vi "User_Metadata.vi"() -> ()   [LabVIEW 2011]
uses:
  ADAM Controls/Channel_names.ctl
  ADAM Controls/Calib_type_ADAM.ctl
  Anemometry/Anemometry Sub Vis/Controls/Preference_Mode.ctl
  ADAM Controls/Channel_State.ctl
  ADAM Controls/Module_type_ADAM.ctl
  ADAM Controls/Update_scan_value.ctl
  Anemometry/Anemometry Sub Vis/Globals/Preference_global.vi
  Anemometry/Anemometry Sub Vis/Globals/Constants_global.vi
  Anemometry/Anemometry Sub Vis/Globals/Meas_global.vi
  Anemometry/Anemometry Sub Vis/Globals/Trav_pos_global.vi
panel:
  out "Channel Name 13":string
  out "Channel Name 12":string
  out "Channel Name 11":string
  in  "Value 13":string
  in  "Value 12":string
  in  "Value 11":string
  in  "Menu 13":u16(ring) items=["Edit Strings", "20mm Cubes"]
  in  "Menu 12":u16(ring) items=["Edit Strings", "20mm Cubes"]
  in  "Menu 11":u16(ring) items=["Edit Strings", "20mm Cubes"]
  in  "Edit Preference Panel":bool
  out "Rig Name":string="EnFlo Tunnel"
  in  "Edit Email Addresses":bool
  out "Email Addresses":string[](array[string])
  in  "Value 10":string
  in  "Value 9":string
  in  "Value 8":string
  in  "Value 7":string
  in  "Value 6":string
  in  "Menu 10":u16(ring) items=["Edit Strings", "20mm Cubes"]
  out "Channel Name 10":string
  in  "Menu 9":u16(ring) items=["Edit Strings", "None", "Ramp 29 x 390mm", "Ramp 9 x 175mm", "Rounded nose 18.2 x 55mm", "Rounded nose 9 x 150mm"]
  out "Channel Name 9":string
  in  "Menu 8":u16(ring) items=["Edit Strings", "20mm Cubes"]
  out "Channel Name 8":string
  in  "Menu 7":u16(ring) items=["Edit Strings", "0", "115", "65"]
  out "Channel Name 7":string
  in  "Menu 6":u16(ring) items=["Edit Strings", "0", "1", "16"]
  out "Channel Name 6":string
  out "Clear remaining channels":bool
  in  "Value 5":string
  in  "Menu 5":u16(ring) items=["Edit Strings", "0", "25", "6.25"]
  out "Channel Name 5":string
  in  "Value 4":string
  in  "Menu 4":u16(ring) items=["Edit Strings", "20 x 20mm", "40 x 40mm", "80 x 80mm", "None"]
  out "Channel Name 4":string
  in  "Value 3":string
  in  "Menu 3":u16(ring) items=["Edit Strings", "0", "10", "20", "Normal distribution with average = 10mm"]
  out "Channel Name 3":string
  in  "Value 2":string
  in  "Menu 2":u16(ring) items=["Edit Strings", "None", "Random blocks", "Uniform cube"]
  out "Channel Name 2":string
  in  "Modify User Channels":bool
  out "Channel No":i32
  out "First Loop":bool
  out "Index":i32
  in  "Value 1":string
  in  "Menu 1":u16(ring) items=["Edit Strings", "Aligned", "None", "Staggered"]
  out "Channel Name 1":string
  in  "stop":bool
  in  "OK":bool
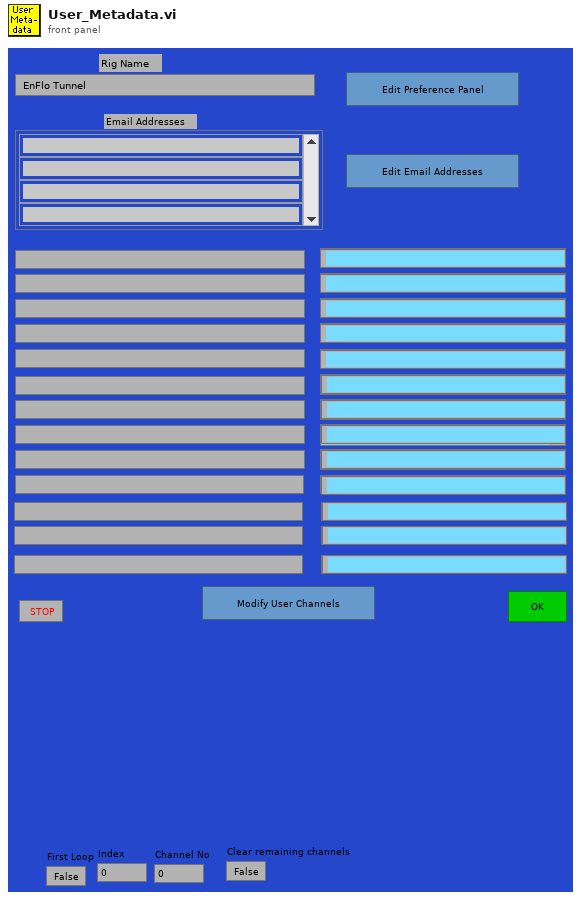
[diagram p1: front panel]
types:
  T1 = typedef "Channel_names.ctl" = enum16{"Active Only", "Active + Off", "All Channels"}
  T2 = typedef "Calib_type_ADAM.ctl" = enum16{"Raw", "Bx + A", "Cx^2 + Bx + A", "Dx^3 + Cx^2 + Bx + A", "In Band", "Hi-Tec Q", "Hi-Tec M_dot", "Text"}
  T3 = typedef "Preference_Mode.ctl" = enum16{"Load Preferences from file", "Save Preferences to file", "Load, Edit then Save"}
  T4 = typedef "Channel_State.ctl" = enum16{"On", "Off", "Always On", "Always Off"}
  T5 = typedef "Module_type_ADAM.ctl" = enum16{"4011", "4012", "4013", "4014", "4016", "4017", "4018", "4021", "4050", "4052", "4053", "4060", "4080", "5000", "5017", "5018", "5024", "5051", "5056", "5060", "6060", "Tracker", "WEST", "GILL", "JEM", "VICI", "Vaisala", "DRUCK", "Run VI Named:", "IR2100", "PPT", "Comparator", "VIRTUAL", "Hold Value", "Read A", "Read Ch", "Coded", "Client Info", "Web Client", "X10", "Test"}
  T6 = typedef "Ch_description_ADAM.ctl" = cluster{"Ch Name":string, "Type":T5, "Function":T7, "Ch State":T4, "Calibration type":T2, "A":dbl, "B":dbl, "C":dbl, "D":dbl, "Comments":string, "Address":T8, "String":string, "Duty":u16}
  T7 = typedef "Function_ADAM.ctl" = enum16{"Analogue Input", "Digital Input", "Event counter", "Event rate", "Analogue Output", "Digital Output", "Relay Output"}
  T8 = typedef "Address.ctl" = cluster{"Main":i32, "Ch.":i32, "Sub":i32, "Port Name":string}
  T9 = typedef "Update_scan_value.ctl" = cluster{"Channel Name":string, "New Value":dbl}
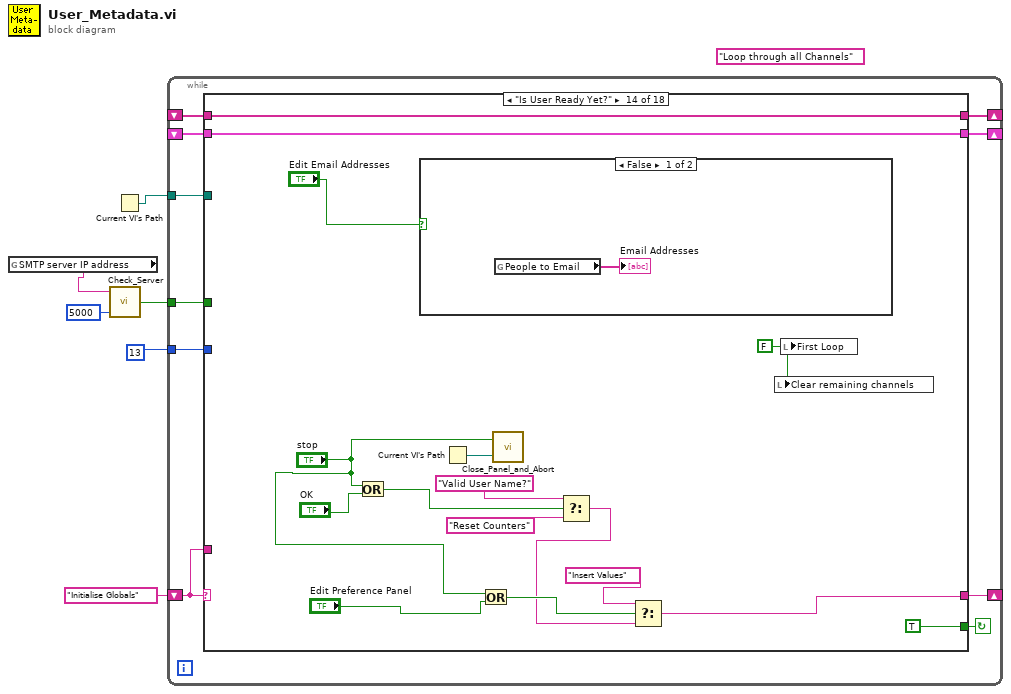
[diagram p0: block diagram]
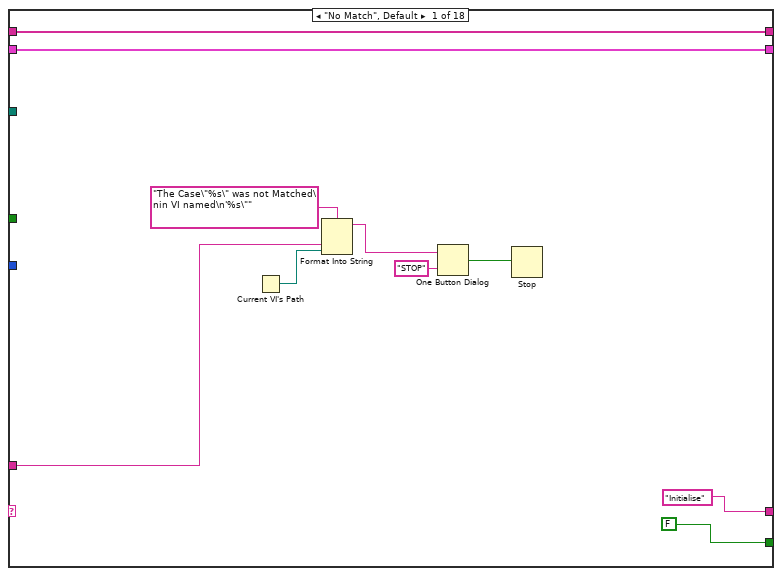
[diagram p2: hidden frame]
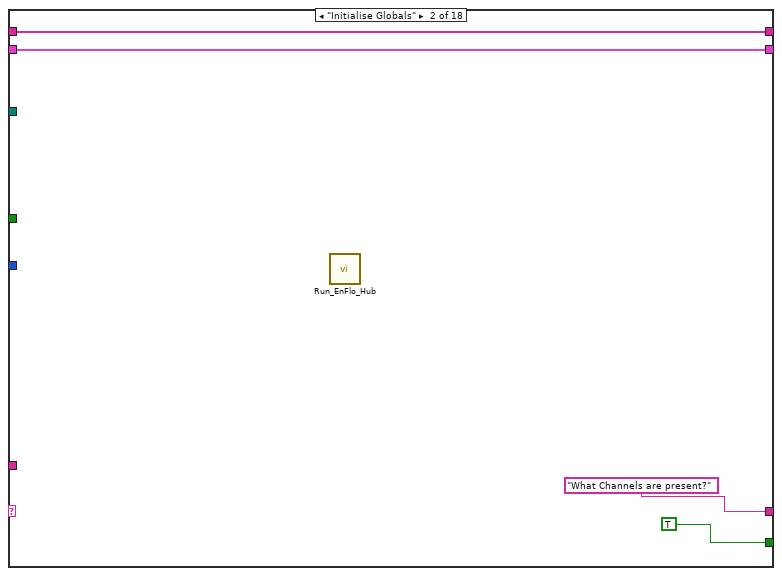
[diagram p3: hidden frame]
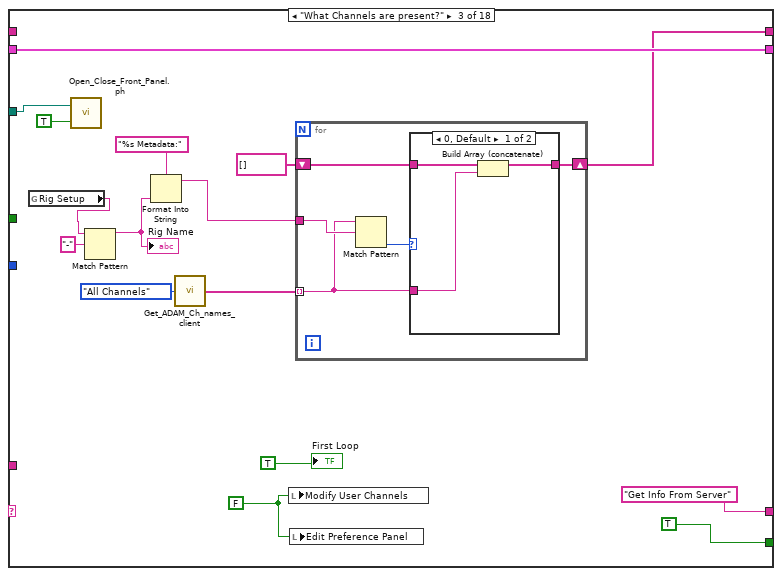
[diagram p4: hidden frame]
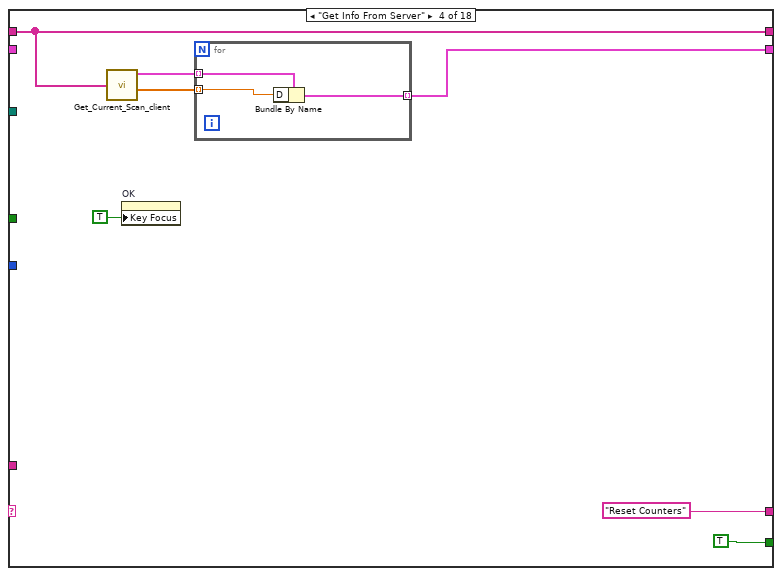
[diagram p6: hidden frame]
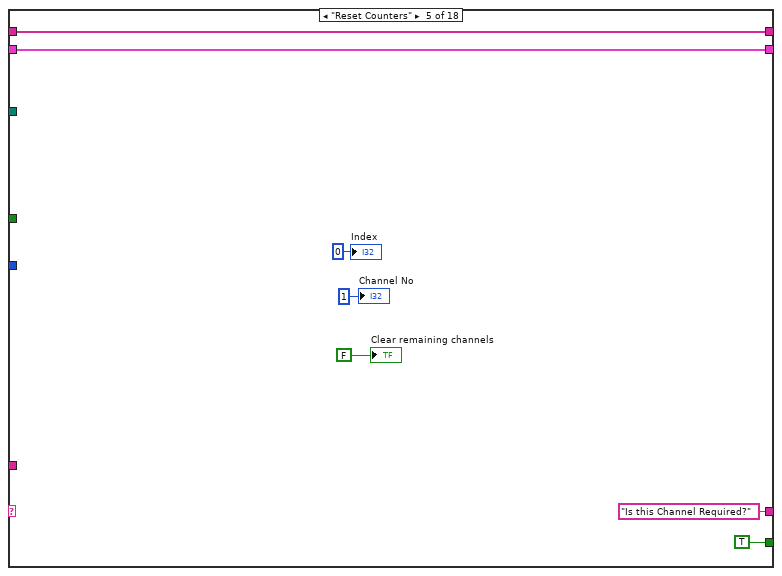
[diagram p7: hidden frame]
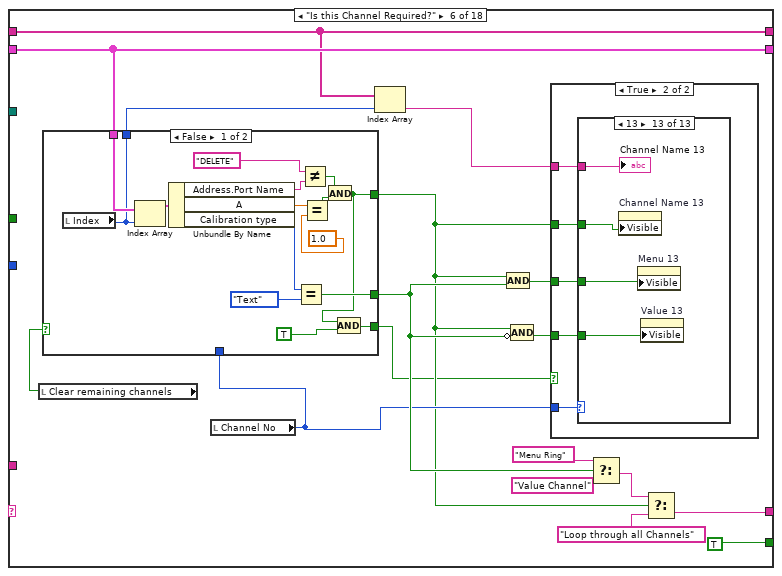
[diagram p8: hidden frame]
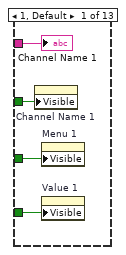
[diagram p10: hidden frame]
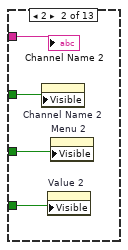
[diagram p11: hidden frame]
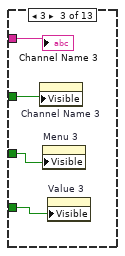
[diagram p12: hidden frame]
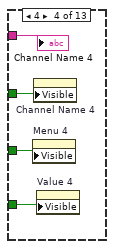
[diagram p13: hidden frame]
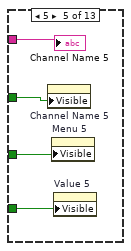
[diagram p14: hidden frame]
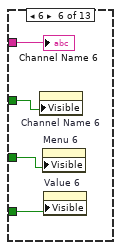
[diagram p15: hidden frame]
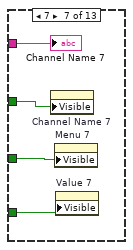
[diagram p16: hidden frame]
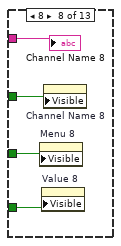
[diagram p17: hidden frame]
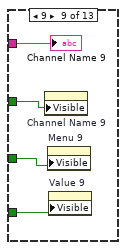
[diagram p18: hidden frame]
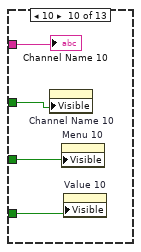
[diagram p19: hidden frame]
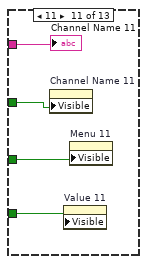
[diagram p20: hidden frame]
diagram:
  (unwired) "Loop through all Channels"
  n1 = global read "Preference_global.vi" "SMTP server IP address"() -> (w2:string)
  n2 = call "Check_Server.vi"("timeout ms (60000)"=5000, "address"=w2) -> ("OK"=w1:bool)  [unwired: 3 out]
  n3 = Current VI's Path() -> (path=w4:path)
  n4 = while {
    tunnel: 13 -> [w9]
    shift-left: _ -> [w12]
    shift-right: [w11] -> _
    shift-left: _ -> [w13]
    shift-right: [w14] -> _
    shift-left: "Initialise Globals" -> [w15]
    shift-right: [w10] -> _
    tunnel: w4 -> [w8]
    tunnel: w1 -> [w7]
    stop <- w16 continue-if-true
    n5 = case shown="\"Is User Ready Yet?\"" w15 {
      tunnel: [FALSE TRUE TRUE TRUE TRUE ("T button?") TRUE TRUE TRUE TRUE TRUE TRUE TRUE TRUE TRUE ("T button?") TRUE ("T button?") TRUE ("T button?") TRUE ("T button?") FALSE ("T button?")] -> w16
      tunnel: ["Initialise" "What Channels are present?" "Get Info From Server" "Reset Counters" "Is this Channel Required?" w84 w178 "Increment Channel No" "Increment Channel No" "Loop through all Channels" w398 "What Channels are present?" "Reset Counters" w447 "Insert Values" "Update Server" w489 "End"] -> w10
      tunnel: w15 -> [w21 _ _ _ _ _ _ _ _ _ _ _ _ _ _ _ _ _]
      tunnel: [w18 w28 w44 w57 w69 w88 w170 w305 w326 w396 w409 w430 w435 w457 w469 w477 w490 w537] -> w14
      tunnel: w13 -> [w18 w28 w44 _ w69 w88 w171 w304 w327 w396 w409 w430 w436 w457 w469 w475 w490 w537]
      tunnel: w12 -> [w17 w27 _ w60 w70 w78 w190 w309 w337 w395 w414 w431 _ w450 w467 w476 w491 w538]
      tunnel: [w17 w27 w40 w60 w70 w78 w190 w309 w337 w395 w414 w431 w434 w450 w467 w476 w491 w538] -> w11
      tunnel: w9 -> [_ _ _ _ _ _ _ _ _ _ w404 _ _ _ _ _ _ _]
      tunnel: w8 -> [_ _ w35 _ _ _ _ _ _ _ _ _ _ _ _ _ _ w535]
      tunnel: w7 -> [_ _ _ _ _ _ _ _ _ _ _ _ _ _ w462 _ _ _]
      frame "No Match", Default {
        n6 = Current VI's Path() -> (path=w20:path)
        n7 = Format Into String(format string="The Case\"%s\" was not Matched\nin VI named\n'%s\"" ("Format String"), w21, w20) -> (resulting string=w24:string)  [unwired: 2 in, 1 out]
        n8 = One Button Dialog(message=w24, button name ("OK")="STOP") -> (true=w22:bool)
        n9 = Stop(stop? (T)=w22) -> ()
      }
      frame "Initialise Globals" {
        n10 = call "Run_EnFlo_Hub.vi"() -> ()  [unwired: 8 out]
      }
      frame "What Channels are present?" {
        w34 = FALSE ("Add a New Channel")
        n11 = global read "Preference_global.vi" "Rig Setup"() -> (w32:string)
        n12 = call "Open_Close_Front_Panel.ph.vi"("Front Panel Window:Open"=TRUE, "VI path"=w35) -> ()  [unwired: 2 out]
        n13 = Match Pattern(string=w32, regular expression="-") -> (before substring=w31:string)  [unwired: 4 out]
        "Rig Name" <- w31
        n14 = Format Into String(format string="%s Metadata:" ("Format String"), w31) -> (resulting string=w37:string)  [unwired: 2 in, 1 out]
        n15 = call "Get_ADAM_Ch_names_client.vi"("Channel names set"=Channel_names."All Channels") -> ("Ch names"=w42:string[])
        n16 = local write "Modify User Channels"(w34) -> ()
        n17 = local write "Edit Preference Panel"(w34) -> ()
        n18 = for {
          tunnel: w37 -> [w51]
          tunnel: w42 -> [w49] mode=indexing
          shift-right: [w47] -> w40
          shift-left: string[] [] -> [w48]
          n19 = Match Pattern(string=w49, regular expression=w51) -> (offset past match=w50:i32)  [unwired: 4 out]
          n20 = case shown="0, Default" w50 {
            tunnel: w49 -> [w54 _]
            tunnel: w48 -> [w53 w55]
            tunnel: [w52 w55] -> w47
            frame 0, Default {
              n21 = Build Array (concatenate)(w53, w54) -> (w52:string[])
            }
            frame -1 {
            }
          }
        }
        "First Loop" <- TRUE ("First Loop")
      }
      frame "Get Info From Server" {
        n22 = call "Get_Current_Scan_client.vi"("ADAM Ch Names"=w60) -> ("Ch Description Array"=w59:T6[], "Numerical Values"=w58:dbl[])  [unwired: 2 out]
        n23 = property on="OK" class="Bool"("Key Focus"=TRUE) -> ()  [unwired: 2 in, 2 out]
        n24 = for {
          tunnel: w59 -> [w65] mode=indexing
          tunnel: w58 -> [w64] mode=indexing
          tunnel: [w63] -> w57 mode=indexing
          n25 = Bundle By Name(cluster=w65, "D"=w64) -> (w63:T6)
        }
      }
      frame "Reset Counters" {
        "Index" <- 0 ("Index")
        "Channel No" <- 1 ("Channel No")
        "Clear remaining channels" <- FALSE ("Clear remaining channels")
      }
      frame "Is this Channel Required?" {
        n26 = local read "Clear remaining channels"() -> (w76:bool)
        n27 = local read "Channel No"() -> (w75:i32)
        n28 = case shown="False" w76 {
          tunnel: w88 -> [w161 _]
          tunnel: [w147 w166] -> w74
          tunnel: [w157 w166] -> w83
          tunnel: [w156 0 ("Index")] -> w79
          tunnel: w75 -> [_ w163]
          tunnel: [w154 TRUE] -> w73
          frame False {
            n29 = local read "Index"() -> (w156:i32)
            n30 = Index Array(array=w161, index=w156) -> (element=w160:T6)
            n31 = Unbundle By Name(w160) -> ("Address.Port Name"=w151:string, "A"=w153:dbl, "Calibration type"=w158:T2)
            n32 = Equal?(x=w158, y=Calib_type_ADAM."Text" ("Calibration Type")) -> (x = y?=w157:bool)
            n33 = Not Equal?(x="DELETE", y=w151) -> (x != y?=w148:bool)
            n34 = Equal?(x=w153, y=1.0 ("x")) -> (x = y?=w149:bool)
            n35 = And(x=w148, y=w149) -> (x .and. y?=w147:bool)
            n36 = Compound Arithmetic op=AND(w147, TRUE ("Input")) -> (w154:bool)
          }
          frame True {
            w166 = FALSE
            n37 = Increment(x=w163) -> (x+1=w164:i32)
            n38 = local write "Channel No"(w164) -> ()
          }
        }
        n39 = Index Array(array=w78, index=w79) -> (element=w77:string)
        n40 = Compound Arithmetic op=AND(w74, w83) -> (w86:bool)
        n41 = Compound Arithmetic op=AND(w74, invert w83) -> (w87:bool)
        n42 = case shown="True" w73 {
          tunnel: w87 -> [_ w94]
          tunnel: w86 -> [_ w93]
          tunnel: w74 -> [_ w92]
          tunnel: w77 -> [_ w91]
          tunnel: w75 -> [_ w90]
          frame False {
          }
          frame True {
            n43 = case shown="13" w90 {
              tunnel: w92 -> [w96 w100 w104 w108 w112 w117 w121 w125 w129 w133 w138 w142 w146]
              tunnel: w94 -> [w98 w102 w106 w110 w114 w115 w119 w123 w127 w131 w135 w139 w143]
              tunnel: w93 -> [w97 w101 w105 w109 w113 w116 w120 w124 w128 w134 w136 w140 w144]
              tunnel: w91 -> [w95 w99 w103 w107 w111 w118 w122 w126 w130 w132 w137 w141 w145]
              frame 1, Default {
                n44 = property on="Channel Name 1" class="Str"("Visible"=w96) -> ()  [unwired: 2 in, 2 out]
                n45 = property on="Menu 1" class="Ring (strict)"("Visible"=w97) -> ()  [unwired: 2 in, 2 out]
                n46 = property on="Value 1" class="Str"("Visible"=w98) -> ()  [unwired: 2 in, 2 out]
                "Channel Name 1" <- w95
              }
              frame 2 {
                n47 = property on="Channel Name 2" class="Str"("Visible"=w100) -> ()  [unwired: 2 in, 2 out]
                n48 = property on="Value 2" class="Str"("Visible"=w102) -> ()  [unwired: 2 in, 2 out]
                n49 = property on="Menu 2" class="Ring (strict)"("Visible"=w101) -> ()  [unwired: 2 in, 2 out]
                "Channel Name 2" <- w99
              }
              frame 3 {
                n50 = property on="Channel Name 3" class="Str"("Visible"=w104) -> ()  [unwired: 2 in, 2 out]
                n51 = property on="Menu 3" class="Ring (strict)"("Visible"=w105) -> ()  [unwired: 2 in, 2 out]
                n52 = property on="Value 3" class="Str"("Visible"=w106) -> ()  [unwired: 2 in, 2 out]
                "Channel Name 3" <- w103
              }
              frame 4 {
                n53 = property on="Menu 4" class="Ring (strict)"("Visible"=w109) -> ()  [unwired: 2 in, 2 out]
                n54 = property on="Channel Name 4" class="Str"("Visible"=w108) -> ()  [unwired: 2 in, 2 out]
                n55 = property on="Value 4" class="Str"("Visible"=w110) -> ()  [unwired: 2 in, 2 out]
                "Channel Name 4" <- w107
              }
              frame 5 {
                n56 = property on="Channel Name 5" class="Str"("Visible"=w112) -> ()  [unwired: 2 in, 2 out]
                n57 = property on="Menu 5" class="Ring (strict)"("Visible"=w113) -> ()  [unwired: 2 in, 2 out]
                n58 = property on="Value 5" class="Str"("Visible"=w114) -> ()  [unwired: 2 in, 2 out]
                "Channel Name 5" <- w111
              }
              frame 6 {
                n59 = property on="Channel Name 6" class="Str"("Visible"=w117) -> ()  [unwired: 2 in, 2 out]
                n60 = property on="Menu 6" class="Ring (strict)"("Visible"=w116) -> ()  [unwired: 2 in, 2 out]
                n61 = property on="Value 6" class="Str"("Visible"=w115) -> ()  [unwired: 2 in, 2 out]
                "Channel Name 6" <- w118
              }
              frame 7 {
                n62 = property on="Channel Name 7" class="Str"("Visible"=w121) -> ()  [unwired: 2 in, 2 out]
                n63 = property on="Menu 7" class="Ring (strict)"("Visible"=w120) -> ()  [unwired: 2 in, 2 out]
                n64 = property on="Value 7" class="Str"("Visible"=w119) -> ()  [unwired: 2 in, 2 out]
                "Channel Name 7" <- w122
              }
              frame 8 {
                n65 = property on="Menu 8" class="Ring (strict)"("Visible"=w124) -> ()  [unwired: 2 in, 2 out]
                n66 = property on="Value 8" class="Str"("Visible"=w123) -> ()  [unwired: 2 in, 2 out]
                n67 = property on="Channel Name 8" class="Str"("Visible"=w125) -> ()  [unwired: 2 in, 2 out]
                "Channel Name 8" <- w126
              }
              frame 9 {
                n68 = property on="Channel Name 9" class="Str"("Visible"=w129) -> ()  [unwired: 2 in, 2 out]
                n69 = property on="Menu 9" class="Ring (strict)"("Visible"=w128) -> ()  [unwired: 2 in, 2 out]
                n70 = property on="Value 9" class="Str"("Visible"=w127) -> ()  [unwired: 2 in, 2 out]
                "Channel Name 9" <- w130
              }
              frame 10 {
                n71 = property on="Channel Name 10" class="Str"("Visible"=w133) -> ()  [unwired: 2 in, 2 out]
                n72 = property on="Menu 10" class="Ring (strict)"("Visible"=w134) -> ()  [unwired: 2 in, 2 out]
                n73 = property on="Value 10" class="Str"("Visible"=w131) -> ()  [unwired: 2 in, 2 out]
                "Channel Name 10" <- w132
              }
              frame 11 {
                n74 = property on="Channel Name 11" class="Str"("Visible"=w138) -> ()  [unwired: 2 in, 2 out]
                n75 = property on="Value 11" class="Str"("Visible"=w135) -> ()  [unwired: 2 in, 2 out]
                n76 = property on="Menu 11" class="Ring (strict)"("Visible"=w136) -> ()  [unwired: 2 in, 2 out]
                "Channel Name 11" <- w137
              }
              frame 12 {
                n77 = property on="Channel Name 12" class="Str"("Visible"=w142) -> ()  [unwired: 2 in, 2 out]
                n78 = property on="Menu 12" class="Ring (strict)"("Visible"=w140) -> ()  [unwired: 2 in, 2 out]
                n79 = property on="Value 12" class="Str"("Visible"=w139) -> ()  [unwired: 2 in, 2 out]
                "Channel Name 12" <- w141
              }
              frame 13 {
                n80 = property on="Channel Name 13" class="Str"("Visible"=w146) -> ()  [unwired: 2 in, 2 out]
                n81 = property on="Menu 13" class="Ring (strict)"("Visible"=w144) -> ()  [unwired: 2 in, 2 out]
                n82 = property on="Value 13" class="Str"("Visible"=w143) -> ()  [unwired: 2 in, 2 out]
                "Channel Name 13" <- w145
              }
            }
          }
        }
        n83 = Select(t="Menu Ring", s=w83, f="Value Channel") -> (s? t:f=w81:string)
        n84 = Select(t=w81, s=w74, f="Loop through all Channels") -> (s? t:f=w84:string)
      }
      frame "Menu Ring" {
        n85 = local read "First Loop"() -> (w188:bool)
        n86 = local read "Index"() -> (w183:i32)
        n87 = Index Array(array=w171, index=w183) -> (element=w168:T6)
        n88 = Unbundle By Name(w168) -> ("String"=w189:string, "D"=w172:dbl)
        n89 = call "Get_array_values_fr_String.vi"("String Value"=w189) -> ("String array"=w176:string[])  [unwired: 1 out]
        n90 = To Unsigned Word Integer(number=w172) -> (unsigned 16bit integer=w187:u16)
        n91 = local read "Channel No"() -> (w182:i32)
        n92 = Build Array (concatenate)("Edit Strings", w176) -> (w177:string[])
        n93 = Increment(x=w187) -> (x+1=w185:u16)
        n94 = Array Size(array=w176) -> (size(s)=w175:i32)
        n95 = To Unsigned Word Integer(number=w175) -> (unsigned 16bit integer=w174:u16)
        n96 = case shown="13" w182 {
          tunnel: w188 -> [w198 w207 w215 w223 w231 w239 w247 w255 w263 w271 w279 w287 w295]
          tunnel: w185 -> [w197 w206 w214 w222 w230 w238 w246 w254 w262 w270 w278 w286 w294]
          tunnel: [w192 w202 w210 w218 w226 w234 w242 w250 w258 w266 w274 w282 w290] -> w184
          tunnel: w177 -> [w196 w200 w209 w217 w225 w232 w241 w249 w257 w265 w273 w281 w289]
          tunnel: w174 -> [w193 w203 w211 w219 w227 w235 w243 w251 w259 w267 w275 w283 w291]
          frame 1, Default {
            n97 = property on="Menu 1" class="Ring (strict)"("Strings []"=w196) -> ()  [unwired: 2 in, 2 out]
            n98 = Select(t=w197, s=w198, f="Menu 1") -> (s? t:f=w194:u16)
            n99 = Less?(x=w194, y=w193) -> (x < y?=w195:bool)
            n100 = Select(t=w194, s=w195, f=w193) -> (s? t:f=w192:u16)
            n101 = local write "Menu 1"(w192) -> ()
          }
          frame 2 {
            n102 = property on="Menu 2" class="Ring (strict)"("Strings []"=w200) -> ()  [unwired: 2 in, 2 out]
            n103 = Select(t=w206, s=w207, f="Menu 2") -> (s? t:f=w204:u16)
            n104 = Less?(x=w204, y=w203) -> (x < y?=w205:bool)
            n105 = Select(t=w204, s=w205, f=w203) -> (s? t:f=w202:u16)
            n106 = local write "Menu 2"(w202) -> ()
          }
          frame 3 {
            n107 = property on="Menu 3" class="Ring (strict)"("Strings []"=w209) -> ()  [unwired: 2 in, 2 out]
            n108 = Select(t=w214, s=w215, f="Menu 3") -> (s? t:f=w212:u16)
            n109 = Less?(x=w212, y=w211) -> (x < y?=w213:bool)
            n110 = Select(t=w212, s=w213, f=w211) -> (s? t:f=w210:u16)
            n111 = local write "Menu 3"(w210) -> ()
          }
          frame 4 {
            n112 = property on="Menu 4" class="Ring (strict)"("Strings []"=w217) -> ()  [unwired: 2 in, 2 out]
            n113 = Select(t=w222, s=w223, f="Menu 4") -> (s? t:f=w220:u16)
            n114 = Less?(x=w220, y=w219) -> (x < y?=w221:bool)
            n115 = Select(t=w220, s=w221, f=w219) -> (s? t:f=w218:u16)
            n116 = local write "Menu 4"(w218) -> ()
          }
          frame 5 {
            n117 = property on="Menu 5" class="Ring (strict)"("Strings []"=w225) -> ()  [unwired: 2 in, 2 out]
            n118 = Select(t=w230, s=w231, f="Menu 5") -> (s? t:f=w228:u16)
            n119 = Less?(x=w228, y=w227) -> (x < y?=w229:bool)
            n120 = Select(t=w228, s=w229, f=w227) -> (s? t:f=w226:u16)
            n121 = local write "Menu 5"(w226) -> ()
          }
          frame 6 {
            n122 = property on="Menu 6" class="Ring (strict)"("Strings []"=w232) -> ()  [unwired: 2 in, 2 out]
            n123 = Select(t=w238, s=w239, f="Menu 6") -> (s? t:f=w236:u16)
            n124 = Less?(x=w236, y=w235) -> (x < y?=w237:bool)
            n125 = Select(t=w236, s=w237, f=w235) -> (s? t:f=w234:u16)
            n126 = local write "Menu 6"(w234) -> ()
          }
          frame 7 {
            n127 = property on="Menu 7" class="Ring (strict)"("Strings []"=w241) -> ()  [unwired: 2 in, 2 out]
            n128 = Select(t=w246, s=w247, f="Menu 7") -> (s? t:f=w244:u16)
            n129 = Less?(x=w244, y=w243) -> (x < y?=w245:bool)
            n130 = Select(t=w244, s=w245, f=w243) -> (s? t:f=w242:u16)
            n131 = local write "Menu 7"(w242) -> ()
          }
          frame 8 {
            n132 = property on="Menu 8" class="Ring (strict)"("Strings []"=w249) -> ()  [unwired: 2 in, 2 out]
            n133 = Select(t=w254, s=w255, f="Menu 8") -> (s? t:f=w252:u16)
            n134 = Less?(x=w252, y=w251) -> (x < y?=w253:bool)
            n135 = Select(t=w252, s=w253, f=w251) -> (s? t:f=w250:u16)
            n136 = local write "Menu 8"(w250) -> ()
          }
          frame 9 {
            n137 = property on="Menu 9" class="Ring (strict)"("Strings []"=w257) -> ()  [unwired: 2 in, 2 out]
            n138 = Select(t=w262, s=w263, f="Menu 9") -> (s? t:f=w260:u16)
            n139 = Less?(x=w260, y=w259) -> (x < y?=w261:bool)
            n140 = Select(t=w260, s=w261, f=w259) -> (s? t:f=w258:u16)
            n141 = local write "Menu 9"(w258) -> ()
          }
          frame 10 {
            n142 = property on="Menu 10" class="Ring (strict)"("Strings []"=w265) -> ()  [unwired: 2 in, 2 out]
            n143 = Select(t=w270, s=w271, f="Menu 10") -> (s? t:f=w268:u16)
            n144 = Less?(x=w268, y=w267) -> (x < y?=w269:bool)
            n145 = Select(t=w268, s=w269, f=w267) -> (s? t:f=w266:u16)
            n146 = local write "Menu 10"(w266) -> ()
          }
          frame 11 {
            n147 = property on="Menu 11" class="Ring (strict)"("Strings []"=w273) -> ()  [unwired: 2 in, 2 out]
            n148 = Select(t=w278, s=w279, f="Menu 11") -> (s? t:f=w276:u16)
            n149 = Less?(x=w276, y=w275) -> (x < y?=w277:bool)
            n150 = Select(t=w276, s=w277, f=w275) -> (s? t:f=w274:u16)
            n151 = local write "Menu 11"(w274) -> ()
          }
          frame 12 {
            n152 = property on="Menu 12" class="Ring (strict)"("Strings []"=w281) -> ()  [unwired: 2 in, 2 out]
            n153 = Select(t=w286, s=w287, f="Menu 12") -> (s? t:f=w284:u16)
            n154 = Less?(x=w284, y=w283) -> (x < y?=w285:bool)
            n155 = Select(t=w284, s=w285, f=w283) -> (s? t:f=w282:u16)
            n156 = local write "Menu 12"(w282) -> ()
          }
          frame 13 {
            n157 = property on="Menu 13" class="Ring (strict)"("Strings []"=w289) -> ()  [unwired: 2 in, 2 out]
            n158 = Select(t=w294, s=w295, f="Menu 13") -> (s? t:f=w292:u16)
            n159 = Less?(x=w292, y=w291) -> (x < y?=w293:bool)
            n160 = Select(t=w292, s=w293, f=w291) -> (s? t:f=w290:u16)
            n161 = local write "Menu 13"(w290) -> ()
          }
        }
        n162 = Equal To 0?(x=w184) -> (x = 0?=w181:bool)
        n163 = Select(t="Edit Menu Strings", s=w181, f="Increment Channel No") -> (s? t:f=w178:string)
        n164 = Decrement(x=w184) -> (x-1=w173:u16)
        n165 = To Double Precision Float(number=w173) -> (double precision float=w169:dbl)
        n166 = Bundle By Name(cluster=w168, "D"=w169) -> (w167:T6)
        n167 = Replace Array Subset(array=w171, new element=w167, index=w183) -> (w170:T6[])
      }
      frame "Edit Menu Strings" {
        n168 = local read "Index"() -> (w299:i32)
        n169 = Index Array(array=w304, index=w299) -> (element=w308:T6)
        n170 = Unbundle By Name(w308) -> ("String"=w310:string, "Ch Name"=w298:string)
        n171 = call "Get_array_values_fr_String.vi"("String Value"=w310) -> ("String array"=w303:string[])  [unwired: 1 out]
        n172 = call "Edit_String_Options_list.vi"("Channel Name"=w298, "String array"=w303) -> ("New Selection Index"=w296:i32, "String array Out"=w302:string[])
        n173 = call "Put_Array_into_String.vi"("String array"=w302) -> ("String Value"=w307:string)
        n174 = local read "Channel No"() -> (w301:i32)
        n175 = Increment(x=w296) -> (x+1=w300:i32)
        n176 = Bundle By Name(cluster=w308, "String"=w307, "D"=w296) -> (w306:T6)
        n177 = To Unsigned Word Integer(number=w300) -> (unsigned 16bit integer=w297:u16)
        n178 = case shown="1, Default" w301 {
          tunnel: w297 -> [w313 w314 w315 w316 w317 w318 w319 w320 w321 w322 w323 w324 w325]
          frame 1, Default {
            n179 = local write "Menu 1"(w313) -> ()
          }
          frame 2 {
            n180 = local write "Menu 2"(w314) -> ()
          }
          frame 3 {
            n181 = local write "Menu 3"(w315) -> ()
          }
          frame 4 {
            n182 = local write "Menu 4"(w316) -> ()
          }
          frame 5 {
            n183 = local write "Menu 5"(w317) -> ()
          }
          frame 6 {
            n184 = local write "Menu 6"(w318) -> ()
          }
          frame 7 {
            n185 = local write "Menu 7"(w319) -> ()
          }
          frame 8 {
            n186 = local write "Menu 8"(w320) -> ()
          }
          frame 9 {
            n187 = local write "Menu 9"(w321) -> ()
          }
          frame 10 {
            n188 = local write "Menu 10"(w322) -> ()
          }
          frame 11 {
            n189 = local write "Menu 11"(w323) -> ()
          }
          frame 12 {
            n190 = local write "Menu 12"(w324) -> ()
          }
          frame 13 {
            n191 = local write "Menu 13"(w325) -> ()
          }
        }
        n192 = Replace Array Subset(array=w304, new element=w306, index=w299) -> (w305:T6[])
      }
      frame "Value Channel" {
        n193 = local read "Index"() -> (w336:i32)
        n194 = local read "First Loop"() -> (w334:bool)
        n195 = Index Array(array=w327, index=w336) -> (element=w328:T6)
        n196 = local read "Channel No"() -> (w335:i32)
        n197 = Unbundle By Name(w328) -> ("D"=w330:dbl)
        n198 = call "Number_2_string.vi"("number"=w330) -> ("String"=w333:string)  [unwired: 1 in]
        n199 = case shown="1, Default" w335 {
          tunnel: w334 -> [w343 w347 w351 w355 w359 w363 w367 w371 w375 w379 w383 w387 w391]
          tunnel: w333 -> [w342 w346 w350 w354 w358 w362 w366 w370 w374 w378 w382 w386 w390]
          tunnel: [w340 w345 w349 w353 w357 w361 w365 w369 w373 w377 w381 w385 w389] -> w332
          frame 1, Default {
            n200 = Select(t=w342, s=w343, f="Value 1") -> (s? t:f=w340:string)
            n201 = local write "Value 1"(w340) -> ()
          }
          frame 2 {
            n202 = Select(t=w346, s=w347, f="Value 2") -> (s? t:f=w345:string)
            n203 = local write "Value 2"(w345) -> ()
          }
          frame 3 {
            n204 = Select(t=w350, s=w351, f="Value 3") -> (s? t:f=w349:string)
            n205 = local write "Value 3"(w349) -> ()
          }
          frame 4 {
            n206 = Select(t=w354, s=w355, f="Value 4") -> (s? t:f=w353:string)
            n207 = local write "Value 4"(w353) -> ()
          }
          frame 5 {
            n208 = Select(t=w358, s=w359, f="Value 5") -> (s? t:f=w357:string)
            n209 = local write "Value 5"(w357) -> ()
          }
          frame 6 {
            n210 = Select(t=w362, s=w363, f="Value 6") -> (s? t:f=w361:string)
            n211 = local write "Value 6"(w361) -> ()
          }
          frame 7 {
            n212 = Select(t=w366, s=w367, f="Value 7") -> (s? t:f=w365:string)
            n213 = local write "Value 7"(w365) -> ()
          }
          frame 8 {
            n214 = Select(t=w370, s=w371, f="Value 8") -> (s? t:f=w369:string)
            n215 = local write "Value 8"(w369) -> ()
          }
          frame 9 {
            n216 = Select(t=w374, s=w375, f="Value 9") -> (s? t:f=w373:string)
            n217 = local write "Value 9"(w373) -> ()
          }
          frame 10 {
            n218 = Select(t=w378, s=w379, f="Value 10") -> (s? t:f=w377:string)
            n219 = local write "Value 10"(w377) -> ()
          }
          frame 11 {
            n220 = Select(t=w382, s=w383, f="Value 11") -> (s? t:f=w381:string)
            n221 = local write "Value 11"(w381) -> ()
          }
          frame 12 {
            n222 = Select(t=w386, s=w387, f="Value 12") -> (s? t:f=w385:string)
            n223 = local write "Value 12"(w385) -> ()
          }
          frame 13 {
            n224 = Select(t=w390, s=w391, f="Value 13") -> (s? t:f=w389:string)
            n225 = local write "Value 13"(w389) -> ()
          }
        }
        n226 = Fract/Exp String To Number(string=w332) -> (number=w331:dbl)  [unwired: 4 out]
        n227 = Bundle By Name(cluster=w328, "D"=w331) -> (w329:T6)
        n228 = Replace Array Subset(array=w327, new element=w329, index=w336) -> (w326:T6[])
      }
      frame "Increment Channel No" {
        n229 = local read "Channel No"() -> (w394:i32)
        n230 = Increment(x=w394) -> (x+1=w393:i32)
        n231 = local write "Channel No"(w393) -> ()
      }
      frame "Loop through all Channels" {
        n232 = local read "Index"() -> (w413:i32)
        n233 = Array Size(array=w409) -> (size(s)=w408:i32)
        n234 = local read "Channel No"() -> (w399:i32)
        n235 = Increment(x=w413) -> (x+1=w412:i32)
        n236 = Less?(x=w412, y=w408) -> (x < y?=w402:bool)
        n237 = local write "Index"(w412) -> ()
        n238 = Less Or Equal?(x=w399, y=w404) -> (x <= y?=w401:bool)
        n239 = Or(x=w402, y=w401) -> (x .or. y?=w403:bool)
        n240 = Compound Arithmetic op=AND(invert w402, w401) -> (w400:bool)
        n241 = case shown="False" w400 {
          frame False {
          }
          frame True {
            n242 = local write "Clear remaining channels"(TRUE ("Clear remaining channels")) -> ()
          }
        }
        n243 = Select(t="Is this Channel Required?", s=w403, f="Is User Ready Yet?") -> (s? t:f=w405:string)
        n244 = Select(t="Edit User Channels", s="Modify User Channels", f=w405) -> (s? t:f=w398:string)
      }
      frame "Edit Preference Panel" {
        n245 = global read "Constants_global.vi" "EnFlo SW Folder"() -> (w418:path)
        n246 = Build Path(base path=w418, name or relative path=path "Anemometry/Utilities/Preference_Panel.vi") -> (appended path=w421:path)
        n247 = Open VI Reference(type specifier VI Refnum (for type only)=refnum<vi> refnum, vi path=w421) -> (vi reference=w428:refnum<vi>, error out=w427:errorcluster)  [unwired: 1 in, 3 out]
        n248 = property class="VI Interface Type 3"(reference=w428, error in=w427, "Front Panel Window:Open"=TRUE) -> (reference out=w425:refnum<vi>, error out=w424:errorcluster)
        n249 = call-by-ref "?"(reference=w425, error in=w424, "Mode"=Preference_Mode."Load, Edit then Save") -> (reference out=w423:refnum<vi>, error out=w422:errorcluster)
        n250 = Close Reference(reference=w423, error in (no error)=w422) -> ()  [unwired: 1 out]
      }
      frame "Edit User Channels" {
        n251 = call "Modify_Metadata_Channels.vi"("Ch Description Array"=w436) -> ("Ch Description Array Out"=w435:T6[])  [unwired: 4 out]
        n252 = local write "First Loop"(TRUE ("First Loop")) -> ()
        n253 = for {
          tunnel: w435 -> [w441] mode=indexing
          tunnel: [w440] -> w434 mode=indexing
          n254 = Unbundle By Name(w441) -> ("Ch Name"=w440:string)
        }
        n255 = local write "Modify User Channels"(FALSE ("Add a New Channel")) -> ()
      }
      frame "Is User Ready Yet?" {
        w449 = FALSE ("First Loop")
        n256 = Or(x="stop", y="OK") -> (x .or. y?=w453:bool)
        n257 = case shown="False" "Edit Email Addresses" {
          frame False {
            n258 = global read "Meas_global.vi" "People to Email"() -> (→"Email Addresses":string[])
          }
          frame True {
            w459 = FALSE  # OK
            n259 = call "Get_users_email_addresses.vi"("OK"=w459) -> ()  [unwired: 5 out]
            n260 = local write "Edit Email Addresses"(FALSE ("Edit Email Addresses")) -> ()
          }
        }
        n261 = Current VI's Path() -> (path=w455:path)
        n262 = Or(x="stop", y="Edit Preference Panel") -> (x .or. y?=w443:bool)
        n263 = call "Close_Panel_and_Abort.vi"("Vi path"=w455, "stop"="stop") -> ()  [unwired: 1 out]
        n264 = Select(t="Valid User Name?", s=w453, f="Reset Counters") -> (s? t:f=w442:string)
        n265 = Select(t="Insert Values", s=w443, f=w442) -> (s? t:f=w447:string)
        n266 = local write "Clear remaining channels"(w449) -> ()
        n267 = local write "First Loop"(w449) -> ()
      }
      frame "Valid User Name?" {
        n268 = local read "Email Addresses"() -> (w466:string[])
        n269 = Array Size(array=w466) -> (size(s)=w465:i32)
        n270 = Equal To 0?(x=w465) -> (x = 0?=w463:bool)
        n271 = And(x=w462, y=w463) -> (x .and. y?=w464:bool)
        n272 = case shown="True" w464 {
          frame False {
          }
          frame True {
            n273 = Two Button Dialog(message="Are you sure you don't want to enter an email address?", 1:"Don't bother" ("F button name (\"Cancel\")"), 2:"Edit Email list" ("T button name (\"OK\")")) -> (T button?=w470:bool)
            n274 = case shown="True" w470 {
              frame False {
              }
              frame True {
                w474 = FALSE  # OK
                n275 = call "Get_users_email_addresses.vi"("OK"=w474) -> ()  [unwired: 5 out]
              }
            }
          }
        }
      }
      frame "Insert Values" {
        n276 = for {
          tunnel: w475 -> [w486] mode=indexing
          tunnel: [w480] -> w477 mode=indexing
          n277 = Unbundle By Name(w486) -> ("A"=w488:dbl)
          n278 = Equal?(x=1.0, y=w488) -> (x = y?=w484:bool)
          n279 = Select(t=Channel_State."On" ("Channel State"), s=w484, f=Channel_State."Off" ("Channel State")) -> (s? t:f=w481:T4)
          n280 = Bundle By Name(cluster=w486, "Type"=Module_type_ADAM."Hold Value" ("Module Type"), "Ch State"=w481) -> (w480:T6)
        }
      }
      frame "Update Server" {
        n281 = stacked-sequence {
          seq-local: [w495 _] -> [_ _]
          seq-local: [w493 _] -> [_ _]
          tunnel: w490 -> [w501 _]
          tunnel: [_ w530] -> w489
          frame #0 {
            w499 = T9 {"Channel Name"="", "New Value"=0.0} ("Update Scan Value Cluster")
            n282 = call "Update_Ch_Discription_client.vi"("Channels to update In"=w501) -> ()  [unwired: 1 out]
            n283 = Initialize Array(w499, 0 ("dimension size")) -> (w500:T9[])
            n284 = for {
              tunnel: w499 -> [w515]
              tunnel: w501 -> [w514] mode=indexing
              shift-right: [w507] -> w497
              shift-left: w500 -> [w508]
              shift-right: [w504] -> w495
              shift-left: i32[] [] -> [w505]
              shift-right: [w502] -> w493
              shift-left: dbl[] [] -> [w503]
              i -> [w506]
              n285 = Unbundle By Name(w514) -> ("Address.Port Name"=w511:string, "Ch Name"=w512:string, "D"=w513:dbl)
              n286 = Not Equal?(x="DELETE", y=w511) -> (x != y?=w509:bool)
              n287 = case shown="True" w509 {
                tunnel: w515 -> [_ w529]
                tunnel: w513 -> [_ w521]
                tunnel: w512 -> [_ w528]
                tunnel: w508 -> [w518 w527]
                tunnel: [w518 w526] -> w507
                tunnel: w506 -> [_ w524]
                tunnel: w505 -> [w517 w523]
                tunnel: [w517 w522] -> w504
                tunnel: w503 -> [w516 w520]
                tunnel: [w516 w519] -> w502
                frame False {
                }
                frame True {
                  n288 = Bundle By Name(cluster=w529, "Channel Name"=w528, "New Value"=w521) -> (w525:T9)
                  n289 = Build Array (concatenate)(w527, w525) -> (w526:T9[])
                  n290 = Build Array (concatenate)(w523, w524) -> (w522:i32[])
                  n291 = Build Array (concatenate)(w520, w521) -> (w519:dbl[])
                }
              }
            }
            n292 = call "Update_Current_Value_client.vi"("Update array in"=w497) -> ()  [unwired: 1 in]
          }
          frame #1 {
            n293 = local read "Edit Preference Panel"() -> (w533:bool)
            n294 = Select(t="Edit Preference Panel", s=w533, f="Close Panel") -> (s? t:f=w530:string)
          }
        }
      }
      frame "Close Panel" {
        n295 = call "Open_Close_Front_Panel.ph.vi"("Front Panel Window:Open"=FALSE, "VI path"=w535) -> ()  [unwired: 2 out]
        n296 = global write "Trav_pos_global.vi" "Show User Metadata on Launch?"(FALSE) -> ()
      }
    }
  }
